vi "SysDef.Create.vi"(8 "error in (no error)":errorcluster, 10 "Diagnostics Configuration":T1={"Interface"="", "Baud Rate"=0, "Diagnostic Protocol"=enum."GMLAN", "Transport Protocol"=enum."ISO TP - Normal Mode", "Transmit ID"=0, "Receive ID"=0, "Transmit Extension"=0, "Receive Extension"=0, "Receive UUDT ID"=0, "Enable Stream"=TRUE, "VW TP Channel ID"=0, "Fill Frame"=FALSE, "Fill Byte"=255, "Termination"=FALSE, "LIN Cluster"="ADCS_LIN_database", "NAD"=1, "IO Mode"=0, "Max DLC"=8, "FD Baud Rate"=0, "Timeout"=0} {"IO Mode" items=["CAN 2.0", "CAN FD", "CAN FD+BRS"]; "Fill Byte" format="%.0x"; "VW TP Channel ID" format="%.0x"; "Receive UUDT ID" format="%.0x"; "Receive Extension" format="%.0x"; "Transmit Extension" format="%.0x"; "Receive ID" format="%.0x"; "Transmit ID" format="%.0x"}, 11 "Device Item Ref in":T5 format="%.0x") -> (0 "error out":errorcluster, 3 "Device Item Ref out":T5 format="%.0x")   [LabVIEW 2019, in "Diagnostics Addon System Explorer.lvlib"]
uses:
  Diagnostics Addon System Explorer.lvlib
  <vilib>/NI VeriStand/Custom Device API/Custom Device Item Ref.ctl
  Addon Shared/Types/CAN.ctl
  Addon Shared/Types/CAN.Interface.ctl
  Addon Shared/Types/Protocol.ctl
  Addon Shared/Types/Transport.ctl
  <vilib>/NI VeriStand/Custom Device API/Custom Device Channel.ctl
  <vilib>/NI VeriStand/Custom Device API/Custom Device Channel Type.ctl
  Addon Shared/Types/Command.New.ctl
  Types/FG.Action.ctl
  Addon Shared/Types/Type.ctl
  Addon Shared/SubVIs/Constants.vi
  <vilib>/NI VeriStand/Custom Device API/NI VeriStand - Get Item Property.vi
  <vilib>/NI VeriStand/Custom Device API/Get Item Property (String).vi
  <vilib>/NI VeriStand/Custom Device API/Get Item Property (Variant).vi
  <vilib>/NI VeriStand/Custom Device API/Get Item Property (U32).vi
  <vilib>/NI VeriStand/Custom Device API/Get Item Property (Boolean).vi
  <vilib>/NI/NI VeriStand Advanced SysDef API/SysDef API/SysDef.Property.Set.vi
  <vilib>/NI/NI VeriStand Advanced SysDef API/_SubVIs/SysDef.Property.Set.String.vi
  <vilib>/NI/NI VeriStand Advanced SysDef API/_SubVIs/SysDef.Property.Set.Variant.vi
  <vilib>/NI/NI VeriStand Advanced SysDef API/_SubVIs/SysDef.Property.Set.U32.vi
  <vilib>/NI/NI VeriStand Advanced SysDef API/_SubVIs/SysDef.Property.Set.Boolean.vi
  <vilib>/NI VeriStand/Custom Device API/Custom Device API.lvlib
  Addon Shared/Diagnostics Addon Shared.lvlib
  <vilib>/NI/NI VeriStand Advanced SysDef API/SysDef API/Advanced System Definition.lvlib
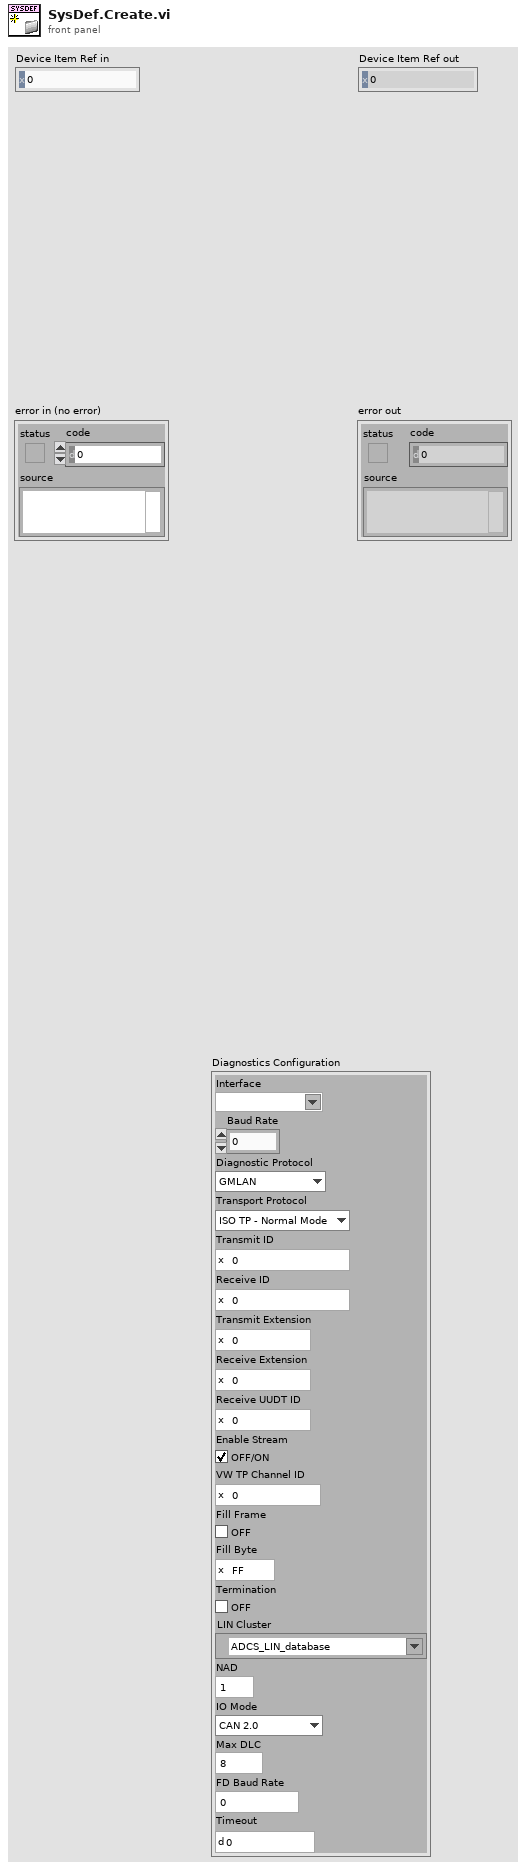
[diagram p1: front panel]
types:
  T1 = typedef "Diagnostics Addon Shared.lvlib/CAN.ctl" = cluster{"Interface":T2, "Baud Rate":u64, "Diagnostic Protocol":T3, "Transport Protocol":T4, "Transmit ID":u32, "Receive ID":u32, "Transmit Extension":u8, "Receive Extension":u8, "Receive UUDT ID":u32, "Enable Stream":bool, "VW TP Channel ID":u32, "Fill Frame":bool, "Fill Byte":u8, "Termination":bool, "LIN Cluster":refnum<k21>, "NAD":u8, "IO Mode":u32, "Max DLC":u16, "FD Baud Rate":u64, "Timeout":u32}
  T2 = typedef "Diagnostics Addon Shared.lvlib/CAN.Interface.ctl" = string
  T3 = typedef "Diagnostics Addon Shared.lvlib/Protocol.ctl" = enum16{"GMLAN", "KWP-2000", "UDS", "User-Defined"}
  T4 = typedef "Diagnostics Addon Shared.lvlib/Transport.ctl" = enum16{"ISO TP - Normal Mode", "ISO TP - Mixed Mode", "VW TP 2.0", "Diagnostics on IP", "ISO TP LIN"}
  T5 = typedef "Custom Device API.lvlib/Custom Device Item Ref.ctl" = u64
  T6 = typedef "Custom Device API.lvlib/Custom Device Channel.ctl" = cluster{"Type":T7, "Units":string, "Default Value":dbl, "Faultable":bool, "Scalable":bool}
  T7 = typedef "Custom Device API.lvlib/Custom Device Channel Type.ctl" = enum16{"Input", "Output"}
  T8 = typedef "Diagnostics Addon Shared.lvlib/Command.New.ctl" = enum8{"None", "Clear Status Channels", "Read All DIDs", "Read All PIDs", "Configure and Start DPIDs", "Stop DPIDs"}
  T9 = typedef "Diagnostics Addon System Explorer.lvlib/FG.Action.ctl" = enum16{"Get", "Set"}
  T10 = typedef "Diagnostics Addon Shared.lvlib/Type.ctl" = enum16{"DID", "CDID", "PID", "CPID", "Read Memory", "Write Memory", "IO Control", "Routine Start", "Routine Request", "Routine Stop", "User Defined", "DTC Control", "Clear DTCs", "Read DTCs", "Start DTCs", "DTC Change Count", "Tester Present", "Unlock ECU", "Reset ECU", "Diag Session Control", "Communication Control", "DPID Control", "Poll Control", "Diag CAN Control"}
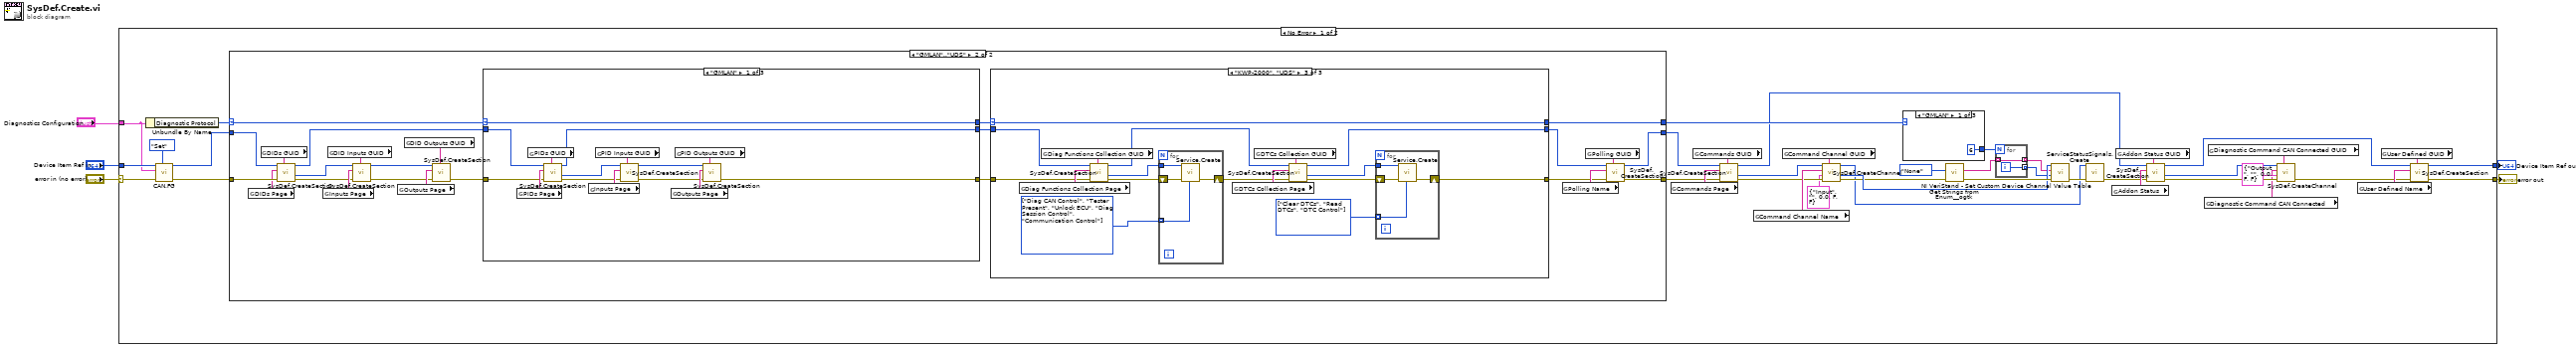
[diagram p0: block diagram]
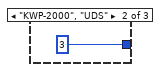
[diagram p2: hidden frame]
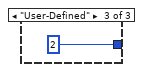
[diagram p3: hidden frame]
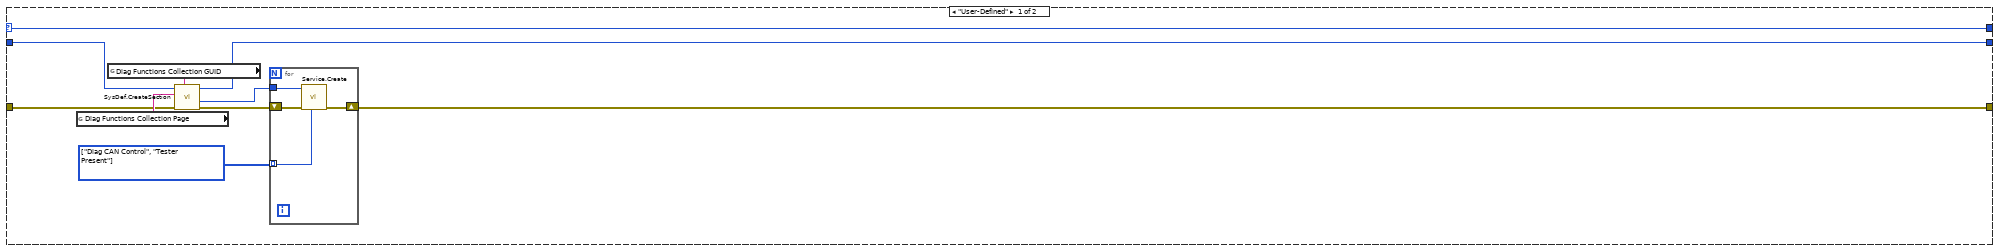
[diagram p4: hidden frame]
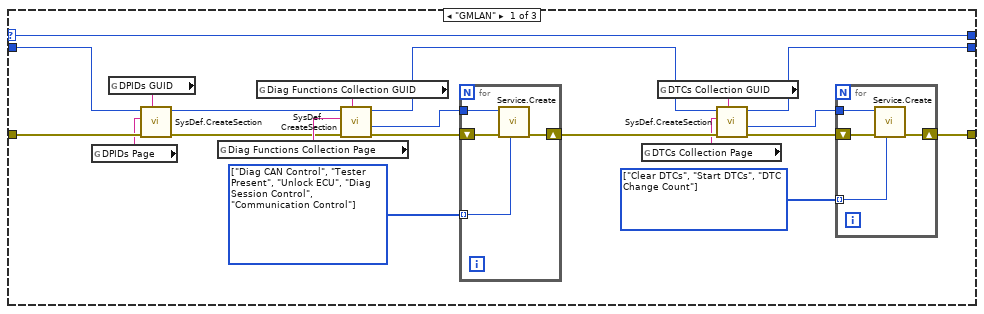
[diagram p5: hidden frame]
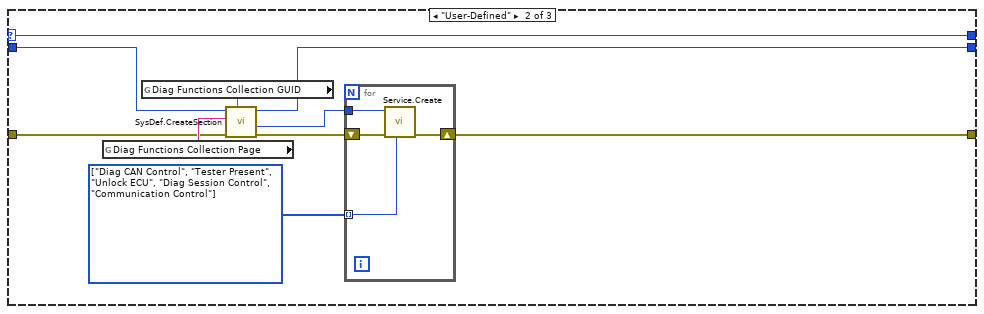
[diagram p6: hidden frame]
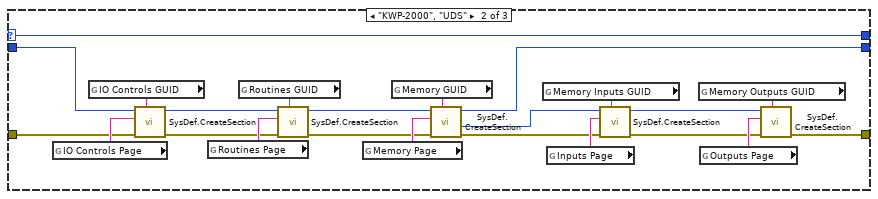
[diagram p7: hidden frame]
diagram:
  n1 = case shown="No Error" "error in (no error)" {
    selector: "error in (no error)" -> [w41 w202]
    tunnel: [w32 w202] -> w4
    tunnel: "Device Item Ref in" -> [w40 w201]
    tunnel: [w33 w201] -> w2
    tunnel: "Diagnostics Configuration" -> [w36 _]
    frame No Error {
      n2 = Unbundle By Name(w36) -> ("Diagnostic Protocol"=w37:T3)
      n3 = call "CAN.FG.vi"("Action"=FG.Action."Set", "error in (no error)"=w41, "Diagnostics Basic Configuration"=w36, "Device Item Ref in"=w40) -> ("error out"=w39:errorcluster, "Device Item Ref out"=w38:T5)  [unwired: 5 in, 1 out]
      n4 = case shown="\"GMLAN\"..\"UDS\"" w37 {
        selector: w37 -> [w62 w75]
        tunnel: w39 -> [w56 w91]
        tunnel: w38 -> [w54 w90]
        tunnel: [w55 w77] -> w20
        tunnel: [w53 w68] -> w21
        tunnel: [w62 w67] -> w22
        frame "User-Defined" {
          w57 = T10[] [enum."Diag CAN Control", enum."Tester Present"] items=["DID", "CDID", "PID", "CPID", "Read Memory", "Write Memory", "IO Control", "Routine Start", "Routine Request", "Routine Stop", "User Defined", "DTC Control", "Clear DTCs", "Read DTCs", "Start DTCs", "DTC Change Count", "Tester Present", "Unlock ECU", "Reset ECU", "Diag Session Control", "Communication Control", "DPID Control", "Poll Control", "Diag CAN Control"]
          n5 = global read "Constants.vi" "Diag Functions Collection Page"() -> (w58:string)
          n6 = global read "Constants.vi" "Diag Functions Collection GUID"() -> (w59:string)
          n7 = call <vilib>:"SysDef.CreateSection.vi"("GUID"=w59, "error in (no error)"=w56, "Name"=w58, "nodeID"=w54) -> ("error out"=w60:errorcluster, "New NodeID"=w61:u64, "nodeID out"=w55:u64)  [unwired: 4 in, 1 out]
          n8 = for {
            tunnel: w61 -> [w65]
            shift-right: [w64] -> w53
            shift-left: w60 -> [w66]
            tunnel: w57 -> [w63] mode=indexing
            n9 = call "Service.Create.vi"("Type"=w63, "error in (no error)"=w66, "Section Ptr"=w65) -> ("error out"=w64:errorcluster)  [unwired: 7 in, 1 out]
          }
        }
        frame "GMLAN".."UDS" {
          n10 = global read "Constants.vi" "DIDs Page"() -> (w89:string)
          n11 = global read "Constants.vi" "DIDs GUID"() -> (w88:string)
          n12 = call <vilib>:"SysDef.CreateSection.vi"("GUID"=w88, "error in (no error)"=w91, "Name"=w89, "nodeID"=w90) -> ("error out"=w85:errorcluster, "New NodeID"=w84:u64, "nodeID out"=w74:u64)  [unwired: 4 in, 1 out]
          n13 = global read "Constants.vi" "Inputs Page"() -> (w86:string)
          n14 = global read "Constants.vi" "DID Inputs GUID"() -> (w87:string)
          n15 = call <vilib>:"SysDef.CreateSection.vi"("GUID"=w87, "error in (no error)"=w85, "Name"=w86, "nodeID"=w84) -> ("error out"=w78:errorcluster, "nodeID out"=w81:u64)  [unwired: 4 in, 2 out]
          n16 = global read "Constants.vi" "Outputs Page"() -> (w82:string)
          n17 = global read "Constants.vi" "DID Outputs GUID"() -> (w83:string)
          n18 = call <vilib>:"SysDef.CreateSection.vi"("GUID"=w83, "error in (no error)"=w78, "Name"=w82, "nodeID"=w81) -> ("error out"=w76:errorcluster)  [unwired: 4 in, 3 out]
          n19 = case shown="\"GMLAN\"" w75 {
            selector: w75 -> [w166 w175 w198]
            tunnel: w76 -> [w168 w180 w200]
            tunnel: w74 -> [w167 w193 w199]
            tunnel: [w165 w188 w199] -> w70
            tunnel: [w160 w176 w200] -> w72
            tunnel: [w166 w175 w198] -> w71
            frame "GMLAN" {
              n20 = global read "Constants.vi" "PIDs Page"() -> (w170:string)
              n21 = global read "Constants.vi" "PIDs GUID"() -> (w169:string)
              n22 = call <vilib>:"SysDef.CreateSection.vi"("GUID"=w169, "error in (no error)"=w168, "Name"=w170, "nodeID"=w167) -> ("error out"=w164:errorcluster, "New NodeID"=w163:u64, "nodeID out"=w165:u64)  [unwired: 4 in, 1 out]
              n23 = global read "Constants.vi" "Inputs Page"() -> (w172:string)
              n24 = global read "Constants.vi" "PID Inputs GUID"() -> (w171:string)
              n25 = call <vilib>:"SysDef.CreateSection.vi"("GUID"=w171, "error in (no error)"=w164, "Name"=w172, "nodeID"=w163) -> ("error out"=w162:errorcluster, "nodeID out"=w161:u64)  [unwired: 4 in, 2 out]
              n26 = global read "Constants.vi" "Outputs Page"() -> (w174:string)
              n27 = global read "Constants.vi" "PID Outputs GUID"() -> (w173:string)
              n28 = call <vilib>:"SysDef.CreateSection.vi"("GUID"=w173, "error in (no error)"=w162, "Name"=w174, "nodeID"=w161) -> ("error out"=w160:errorcluster)  [unwired: 4 in, 3 out]
            }
            frame "KWP-2000", "UDS" {
              n29 = global read "Constants.vi" "IO Controls Page"() -> (w194:string)
              n30 = global read "Constants.vi" "IO Controls GUID"() -> (w195:string)
              n31 = call <vilib>:"SysDef.CreateSection.vi"("GUID"=w195, "error in (no error)"=w180, "Name"=w194, "nodeID"=w193) -> ("error out"=w179:errorcluster, "nodeID out"=w192:u64)  [unwired: 4 in, 2 out]
              n32 = global read "Constants.vi" "Routines Page"() -> (w197:string)
              n33 = global read "Constants.vi" "Routines GUID"() -> (w196:string)
              n34 = call <vilib>:"SysDef.CreateSection.vi"("GUID"=w196, "error in (no error)"=w179, "Name"=w197, "nodeID"=w192) -> ("error out"=w178:errorcluster, "nodeID out"=w189:u64)  [unwired: 4 in, 2 out]
              n35 = global read "Constants.vi" "Memory Page"() -> (w190:string)
              n36 = global read "Constants.vi" "Memory GUID"() -> (w191:string)
              n37 = call <vilib>:"SysDef.CreateSection.vi"("GUID"=w191, "error in (no error)"=w178, "Name"=w190, "nodeID"=w189) -> ("error out"=w182:errorcluster, "New NodeID"=w181:u64, "nodeID out"=w188:u64)  [unwired: 4 in, 1 out]
              n38 = global read "Constants.vi" "Memory Inputs GUID"() -> (w187:string)
              n39 = global read "Constants.vi" "Inputs Page"() -> (w186:string)
              n40 = call <vilib>:"SysDef.CreateSection.vi"("GUID"=w187, "error in (no error)"=w182, "Name"=w186, "nodeID"=w181) -> ("error out"=w177:errorcluster, "nodeID out"=w185:u64)  [unwired: 4 in, 2 out]
              n41 = global read "Constants.vi" "Memory Outputs GUID"() -> (w183:string)
              n42 = global read "Constants.vi" "Outputs Page"() -> (w184:string)
              n43 = call <vilib>:"SysDef.CreateSection.vi"("GUID"=w183, "error in (no error)"=w177, "Name"=w184, "nodeID"=w185) -> ("error out"=w176:errorcluster)  [unwired: 4 in, 3 out]
            }
            frame "User-Defined" {
            }
          }
          n44 = case shown="\"KWP-2000\", \"UDS\"" w71 {
            selector: w71 -> [w92 w121 w135]
            tunnel: [w111 w123 w137] -> w69
            tunnel: [w112 w122 w138] -> w73
            tunnel: w72 -> [w103 w125 w139]
            tunnel: w70 -> [w102 w124 w136]
            tunnel: [w92 w121 w135] -> w67
            frame "GMLAN" {
              w97 = T10[] [enum."Clear DTCs", enum."Start DTCs", enum."DTC Change Count"] items=["DID", "CDID", "PID", "CPID", "Read Memory", "Write Memory", "IO Control", "Routine Start", "Routine Request", "Routine Stop", "User Defined", "DTC Control", "Clear DTCs", "Read DTCs", "Start DTCs", "DTC Change Count", "Tester Present", "Unlock ECU", "Reset ECU", "Diag Session Control", "Communication Control", "DPID Control", "Poll Control", "Diag CAN Control"]
              w98 = T10[] [enum."Diag CAN Control", enum."Tester Present", enum."Unlock ECU", enum."Diag Session Control", enum."Communication Control"] items=["DID", "CDID", "PID", "CPID", "Read Memory", "Write Memory", "IO Control", "Routine Start", "Routine Request", "Routine Stop", "User Defined", "DTC Control", "Clear DTCs", "Read DTCs", "Start DTCs", "DTC Change Count", "Tester Present", "Unlock ECU", "Reset ECU", "Diag Session Control", "Communication Control", "DPID Control", "Poll Control", "Diag CAN Control"]
              n45 = global read "Constants.vi" "DPIDs Page"() -> (w94:string)
              n46 = global read "Constants.vi" "DPIDs GUID"() -> (w93:string)
              n47 = call <vilib>:"SysDef.CreateSection.vi"("GUID"=w93, "error in (no error)"=w103, "Name"=w94, "nodeID"=w102) -> ("error out"=w95:errorcluster, "nodeID out"=w100:u64)  [unwired: 4 in, 2 out]
              n48 = global read "Constants.vi" "Diag Functions Collection Page"() -> (w104:string)
              n49 = global read "Constants.vi" "Diag Functions Collection GUID"() -> (w105:string)
              n50 = call <vilib>:"SysDef.CreateSection.vi"("GUID"=w105, "error in (no error)"=w95, "Name"=w104, "nodeID"=w100) -> ("error out"=w106:errorcluster, "New NodeID"=w107:u64, "nodeID out"=w101:u64)  [unwired: 4 in, 1 out]
              n51 = for {
                tunnel: w107 -> [w115]
                shift-right: [w114] -> w99
                shift-left: w106 -> [w116]
                tunnel: w98 -> [w113] mode=indexing
                n52 = call "Service.Create.vi"("Type"=w113, "error in (no error)"=w116, "Section Ptr"=w115) -> ("error out"=w114:errorcluster)  [unwired: 7 in, 1 out]
              }
              n53 = global read "Constants.vi" "DTCs Collection Page"() -> (w96:string)
              n54 = global read "Constants.vi" "DTCs Collection GUID"() -> (w110:string)
              n55 = call <vilib>:"SysDef.CreateSection.vi"("GUID"=w110, "error in (no error)"=w99, "Name"=w96, "nodeID"=w101) -> ("error out"=w109:errorcluster, "New NodeID"=w108:u64, "nodeID out"=w111:u64)  [unwired: 4 in, 1 out]
              n56 = for {
                tunnel: w108 -> [w119]
                shift-right: [w118] -> w112
                shift-left: w109 -> [w120]
                tunnel: w97 -> [w117] mode=indexing
                n57 = call "Service.Create.vi"("Type"=w117, "error in (no error)"=w120, "Section Ptr"=w119) -> ("error out"=w118:errorcluster)  [unwired: 7 in, 1 out]
              }
            }
            frame "User-Defined" {
              w126 = T10[] [enum."Diag CAN Control", enum."Tester Present", enum."Unlock ECU", enum."Diag Session Control", enum."Communication Control"] items=["DID", "CDID", "PID", "CPID", "Read Memory", "Write Memory", "IO Control", "Routine Start", "Routine Request", "Routine Stop", "User Defined", "DTC Control", "Clear DTCs", "Read DTCs", "Start DTCs", "DTC Change Count", "Tester Present", "Unlock ECU", "Reset ECU", "Diag Session Control", "Communication Control", "DPID Control", "Poll Control", "Diag CAN Control"]
              n58 = global read "Constants.vi" "Diag Functions Collection Page"() -> (w127:string)
              n59 = global read "Constants.vi" "Diag Functions Collection GUID"() -> (w128:string)
              n60 = call <vilib>:"SysDef.CreateSection.vi"("GUID"=w128, "error in (no error)"=w125, "Name"=w127, "nodeID"=w124) -> ("error out"=w129:errorcluster, "New NodeID"=w130:u64, "nodeID out"=w123:u64)  [unwired: 4 in, 1 out]
              n61 = for {
                tunnel: w130 -> [w133]
                shift-right: [w132] -> w122
                shift-left: w129 -> [w134]
                tunnel: w126 -> [w131] mode=indexing
                n62 = call "Service.Create.vi"("Type"=w131, "error in (no error)"=w134, "Section Ptr"=w133) -> ("error out"=w132:errorcluster)  [unwired: 7 in, 1 out]
              }
            }
            frame "KWP-2000", "UDS" {
              w140 = T10[] [enum."Clear DTCs", enum."Read DTCs", enum."DTC Control"] items=["DID", "CDID", "PID", "CPID", "Read Memory", "Write Memory", "IO Control", "Routine Start", "Routine Request", "Routine Stop", "User Defined", "DTC Control", "Clear DTCs", "Read DTCs", "Start DTCs", "DTC Change Count", "Tester Present", "Unlock ECU", "Reset ECU", "Diag Session Control", "Communication Control", "DPID Control", "Poll Control", "Diag CAN Control"]
              w141 = T10[] [enum."Diag CAN Control", enum."Tester Present", enum."Unlock ECU", enum."Diag Session Control", enum."Communication Control"] items=["DID", "CDID", "PID", "CPID", "Read Memory", "Write Memory", "IO Control", "Routine Start", "Routine Request", "Routine Stop", "User Defined", "DTC Control", "Clear DTCs", "Read DTCs", "Start DTCs", "DTC Change Count", "Tester Present", "Unlock ECU", "Reset ECU", "Diag Session Control", "Communication Control", "DPID Control", "Poll Control", "Diag CAN Control"]
              n63 = global read "Constants.vi" "Diag Functions Collection Page"() -> (w144:string)
              n64 = global read "Constants.vi" "Diag Functions Collection GUID"() -> (w145:string)
              n65 = call <vilib>:"SysDef.CreateSection.vi"("GUID"=w145, "error in (no error)"=w139, "Name"=w144, "nodeID"=w136) -> ("error out"=w146:errorcluster, "New NodeID"=w147:u64, "nodeID out"=w143:u64)  [unwired: 4 in, 1 out]
              n66 = for {
                tunnel: w147 -> [w154]
                shift-right: [w153] -> w142
                shift-left: w146 -> [w155]
                tunnel: w141 -> [w152] mode=indexing
                n67 = call "Service.Create.vi"("Type"=w152, "error in (no error)"=w155, "Section Ptr"=w154) -> ("error out"=w153:errorcluster)  [unwired: 7 in, 1 out]
              }
              n68 = global read "Constants.vi" "DTCs Collection Page"() -> (w151:string)
              n69 = global read "Constants.vi" "DTCs Collection GUID"() -> (w150:string)
              n70 = call <vilib>:"SysDef.CreateSection.vi"("GUID"=w150, "error in (no error)"=w142, "Name"=w151, "nodeID"=w143) -> ("error out"=w149:errorcluster, "New NodeID"=w148:u64, "nodeID out"=w137:u64)  [unwired: 4 in, 1 out]
              n71 = for {
                tunnel: w148 -> [w158]
                shift-right: [w157] -> w138
                shift-left: w149 -> [w159]
                tunnel: w140 -> [w156] mode=indexing
                n72 = call "Service.Create.vi"("Type"=w156, "error in (no error)"=w159, "Section Ptr"=w158) -> ("error out"=w157:errorcluster)  [unwired: 7 in, 1 out]
              }
            }
          }
          n73 = global read "Constants.vi" "Polling Name"() -> (w80:string)
          n74 = global read "Constants.vi" "Polling GUID"() -> (w79:string)
          n75 = call <vilib>:"SysDef.CreateSection.vi"("GUID"=w79, "error in (no error)"=w73, "Name"=w80, "nodeID"=w69) -> ("error out"=w68:errorcluster, "nodeID out"=w77:u64)  [unwired: 4 in, 2 out]
        }
      }
      n76 = global read "Constants.vi" "Commands Page"() -> (w47:string)
      n77 = global read "Constants.vi" "Commands GUID"() -> (w46:string)
      n78 = call <vilib>:"SysDef.CreateSection.vi"("GUID"=w46, "error in (no error)"=w21, "Name"=w47, "nodeID"=w20) -> ("error out"=w35:errorcluster, "New NodeID"=w34:u64, "nodeID out"=w13:u64)  [unwired: 4 in, 1 out]
      n79 = global read "Constants.vi" "Command Channel Name"() -> (w42:string)
      n80 = global read "Constants.vi" "Command Channel GUID"() -> (w30:string)
      n81 = call <vilib>:"SysDef.CreateChannel.vi"("GUID"=w30, "error in (no error)"=w35, "Channel"=T6 {"Type"=enum."Input", "Units"="", "Default Value"=0.0, "Faultable"=FALSE, "Scalable"=FALSE}, "Name"=w42, "nodeID"=w34) -> ("error out"=w18:errorcluster, "New NodeID"=w27:u64, "nodeID out"=w17:u64)  [unwired: 3 in, 1 out]
      n82 = case shown="\"GMLAN\"" w22 {
        tunnel: [6 3 2] -> w23
        frame "GMLAN" {
        }
        frame "KWP-2000", "UDS" {
        }
        frame "User-Defined" {
        }
      }
      n83 = call <userlib>:"Get Strings from Enum__ogtk.vi"("error in (no error)"=w18, "Enum"=Command.New."None") -> ("error out"=w28:errorcluster, "Enum Strings"=w26:string[])  [unwired: 6 in, 2 out]
      n84 = for {
        N: w23 -> [_]
        tunnel: w26 -> [w51] mode=indexing
        tunnel: [w52] -> w24 mode=indexing
        tunnel: [w51] -> w25 mode=indexing
        i -> [w52]
      }
      n85 = call <vilib>:"NI VeriStand - Set Custom Device Channel Value Table.vi"("error in (no error)"=w28, "Values"=w24, "Names"=w25, "Channel Ref in"=w27) -> ("error out"=w19:errorcluster)  [unwired: 6 in, 1 out]
      n86 = call "ServiceStatusSignals.Create.vi"("error in (no error)"=w19, "nodeID in"=w17) -> ("error out"=w14:errorcluster)  [unwired: 8 in, 1 out]
      n87 = global read "Constants.vi" "Addon Status"() -> (w16:string)
      n88 = global read "Constants.vi" "Addon Status GUID"() -> (w15:string)
      n89 = call <vilib>:"SysDef.CreateSection.vi"("GUID"=w15, "error in (no error)"=w14, "Name"=w16, "nodeID"=w13) -> ("error out"=w9:errorcluster, "New NodeID"=w10:u64, "nodeID out"=w6:u64)  [unwired: 4 in, 1 out]
      n90 = global read "Constants.vi" "Diagnostic Command CAN Connected"() -> (w7:string)
      n91 = global read "Constants.vi" "Diagnostic Command CAN Connected GUID"() -> (w11:string)
      n92 = call <vilib>:"SysDef.CreateChannel.vi"("GUID"=w11, "error in (no error)"=w9, "Channel"=T6 {"Type"=enum."Output", "Units"="", "Default Value"=0.0, "Faultable"=FALSE, "Scalable"=FALSE}, "Name"=w7, "nodeID"=w10) -> ("error out"=w8:errorcluster)  [unwired: 3 in, 3 out]
      n93 = global read "Constants.vi" "User Defined Name"() -> (w43:string)
      n94 = global read "Constants.vi" "User Defined GUID"() -> (w44:string)
      n95 = call <vilib>:"SysDef.CreateSection.vi"("GUID"=w44, "error in (no error)"=w8, "Name"=w43, "nodeID"=w6) -> ("error out"=w32:errorcluster, "nodeID out"=w33:u64)  [unwired: 4 in, 2 out]
    }
    frame Error {
    }
  }
  "error out" <- w4
  "Device Item Ref out" <- w2
